vi "FGV Messwerte_PMA.vi"(0 "GasValue":sgl[](array[numeric]), 1 "Messbereich":T2 items=["0-500ppm"=1, "0-2500ppm"=2, "0-10000ppm"=3], 4 "Zielmessbereich":u16, 7 "Prüfgaskonz.":sgl, 8 "Kalibrieren":T4, 9 "Aktion":T5=enum."Messen", 13 "CAL-Daten Tolernaz":T1) -> (14 "Rohwerte LIN":sgl[](array[numeric]), 16 "Rohwerte":sgl[](array[numeric]), 19 "im gültigen Bereich":bool, 20 "GasValue":sgl[](array[numeric]), 21 "CAL-Daten":T3={"O2 Null"=0.0, "O2 Steil"=[1.0, 1.0, 1.0, 1.0]}, 24 "CAL-Daten Tolernaz":T1, 25 "Kalibrieren erfolgreich":bool, 27 "CAL TimeOut":bool)   [LabVIEW 2020, in "ABB-EL3000.lvlib" / "PMA.lvlib" / "Kalibrieren.lvlib"]
uses:
  Kalibrieren.lvlib
  Allgemeine VI/FGV Uras26 Aktion.ctl
  Kalibrierung O2.ctl
  Allgemeine VI/CAL-Daten PMA.ctl
  Allgemeine VI/Messbereich CO lo.ctl
  Allgemeine VI/CAL-Daten Toleranz.ctl
  Auto Kalibrieren/KAL Daten loggen Aktionen.ctl
  Allgemeine VI/Aktionen Cal Daten speichern.ctl
  Allgemein/allgemeine Sub-VIs.lvlib
  Allgemeine VI/Allgemeine VI.lvlib
  Auto Kalibrieren/Auto Kalibrieren.lvlib
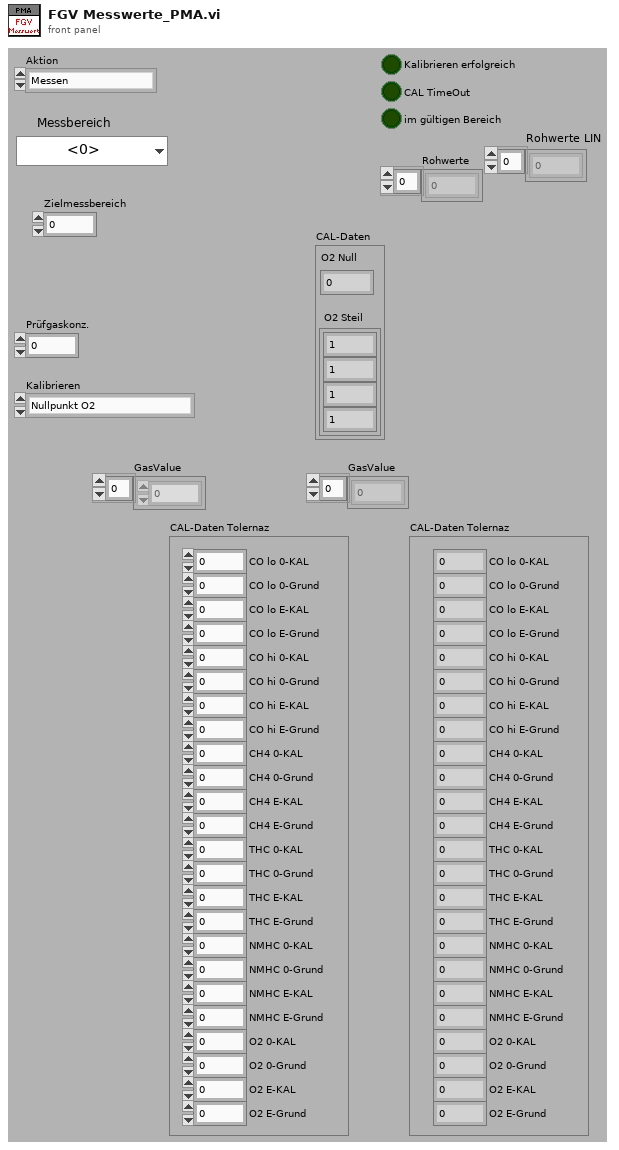
[diagram p1: front panel]
types:
  T1 = typedef "ABB-EL3000.lvlib/Allgemeine VI.lvlib/CAL-Daten Toleranz.ctl" = cluster{"CO lo 0-KAL":sgl, "CO lo 0-Grund":sgl, "CO lo E-KAL":sgl, "CO lo E-Grund":sgl, "CO hi 0-KAL":sgl, "CO hi 0-Grund":sgl, "CO hi E-KAL":sgl, "CO hi E-Grund":sgl, "CH4 0-KAL":sgl, "CH4 0-Grund":sgl, "CH4 E-KAL":sgl, "CH4 E-Grund":sgl, "THC 0-KAL":sgl, "THC 0-Grund":sgl, "THC E-KAL":sgl, "THC E-Grund":sgl, "NMHC 0-KAL":sgl, "NMHC 0-Grund":sgl, "NMHC E-KAL":sgl, "NMHC E-Grund":sgl, "O2 0-KAL":sgl, "O2 0-Grund":sgl, "O2 E-KAL":sgl, "O2 E-Grund":sgl}
  T2 = typedef "ABB-EL3000.lvlib/Allgemeine VI.lvlib/Messbereich CO lo.ctl" = u16
  T3 = typedef "ABB-EL3000.lvlib/Allgemeine VI.lvlib/CAL-Daten PMA.ctl" = cluster{"O2 Null":sgl, "O2 Steil":sgl[]}
  T4 = typedef "ABB-EL3000.lvlib/PMA.lvlib/Kalibrieren.lvlib/Kalibrierung O2.ctl" = enum16{"Nullpunkt O2", "Endpunkt O2"}
  T5 = typedef "ABB-EL3000.lvlib/Allgemeine VI.lvlib/FGV Uras26 Aktion.ctl" = enum16{"lesen", "CAL-Daten laden", "Messen", "Kalibrieren vorbereiten", "Kalibrieren", "CAL-Daten speichern", "Toleranz schreiben", "CAL-Daten kopieren"}
  T6 = typedef "Auto Kalibrieren.lvlib/KAL Daten loggen Aktionen.ctl" = enum16{"lesen", "initialisieren", "loggen"}
  T7 = typedef "ABB-EL3000.lvlib/Allgemeine VI.lvlib/Aktionen Cal Daten speichern.ctl" = enum16{"Cal Daten", "Toleranzen", "PMA", "FID", "Cal Daten PMA", "Cal Daten FID"}
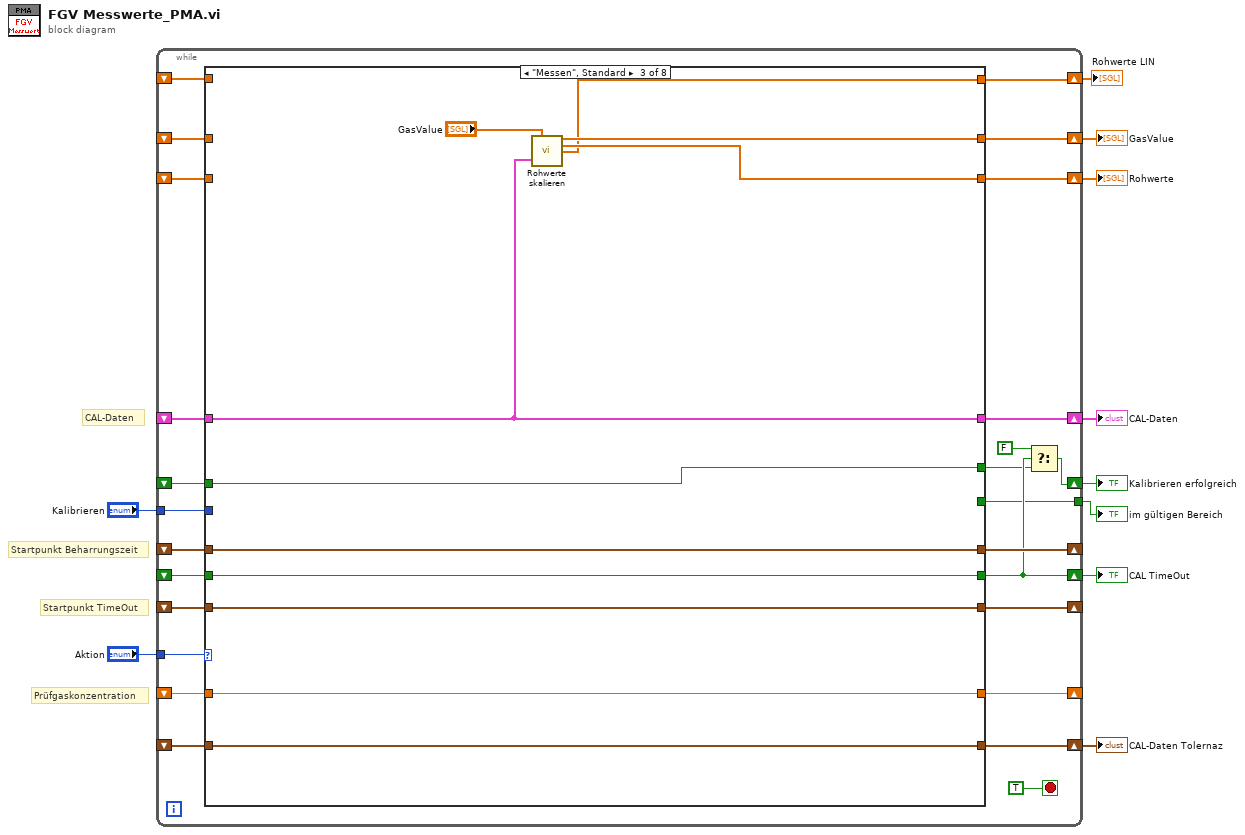
[diagram p0: block diagram]
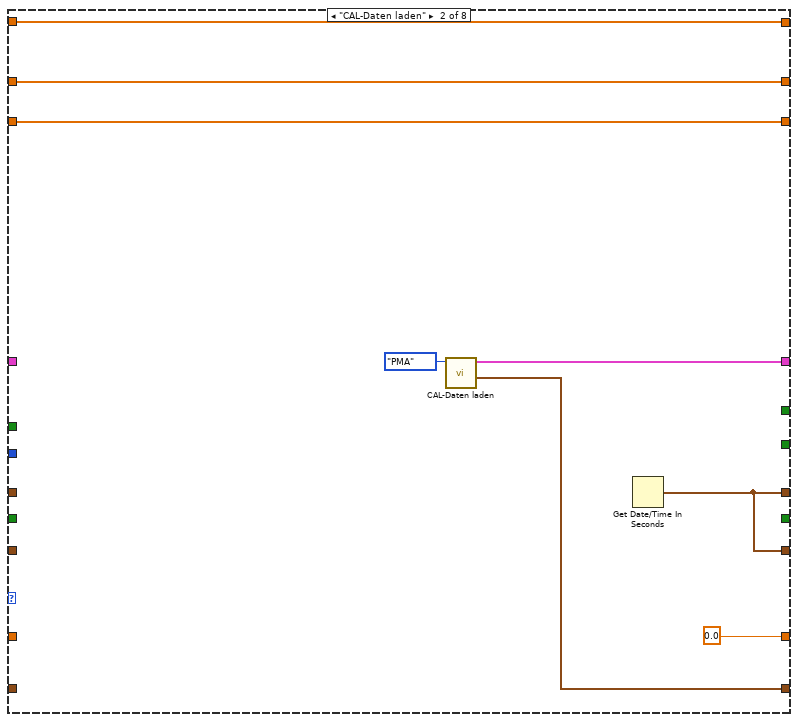
[diagram p3: hidden frame]
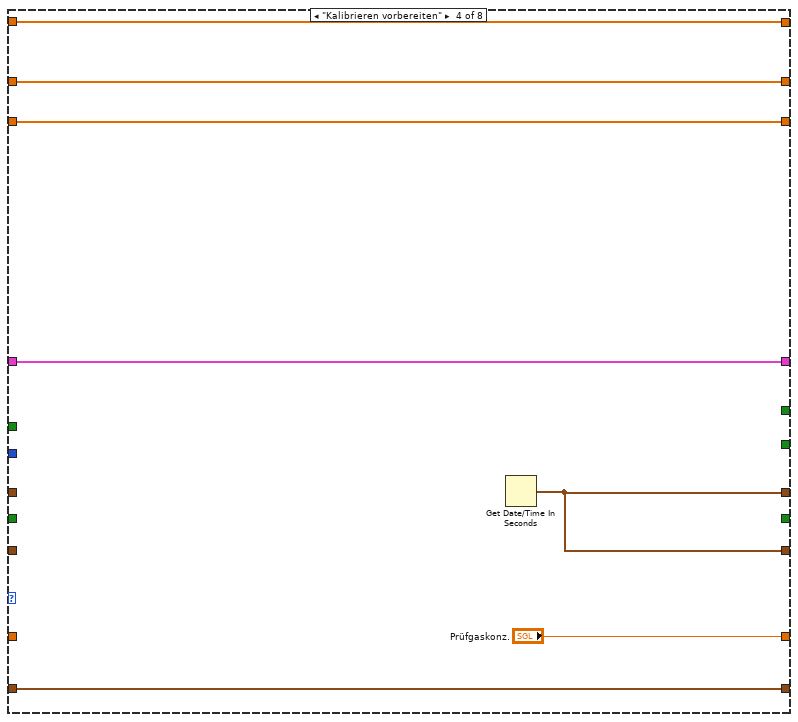
[diagram p4: hidden frame]
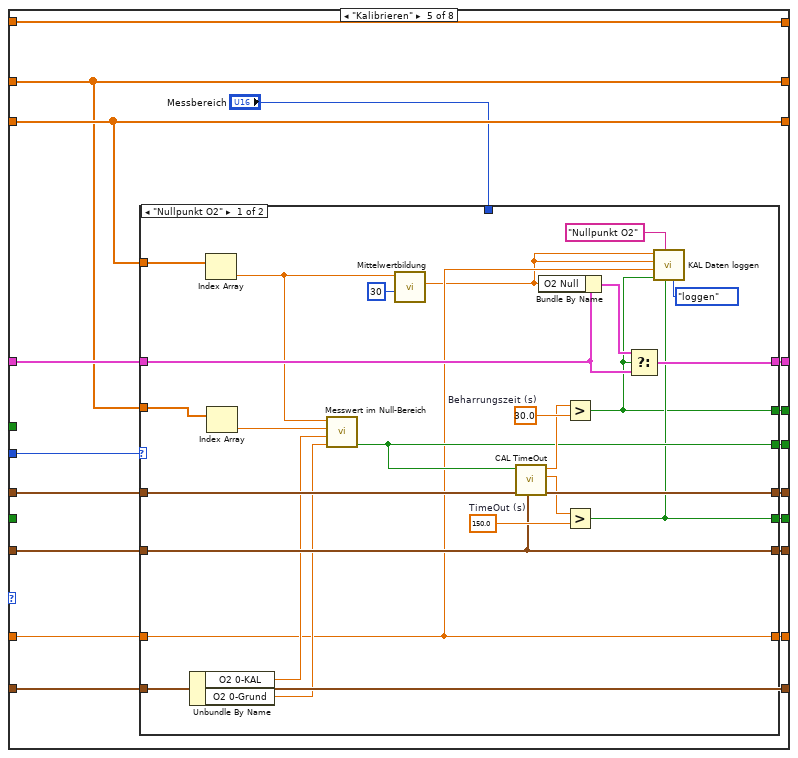
[diagram p5: hidden frame]
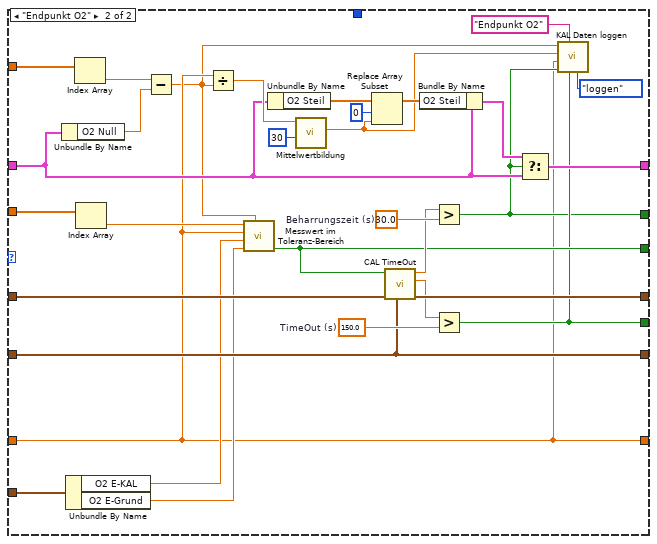
[diagram p6: hidden frame]
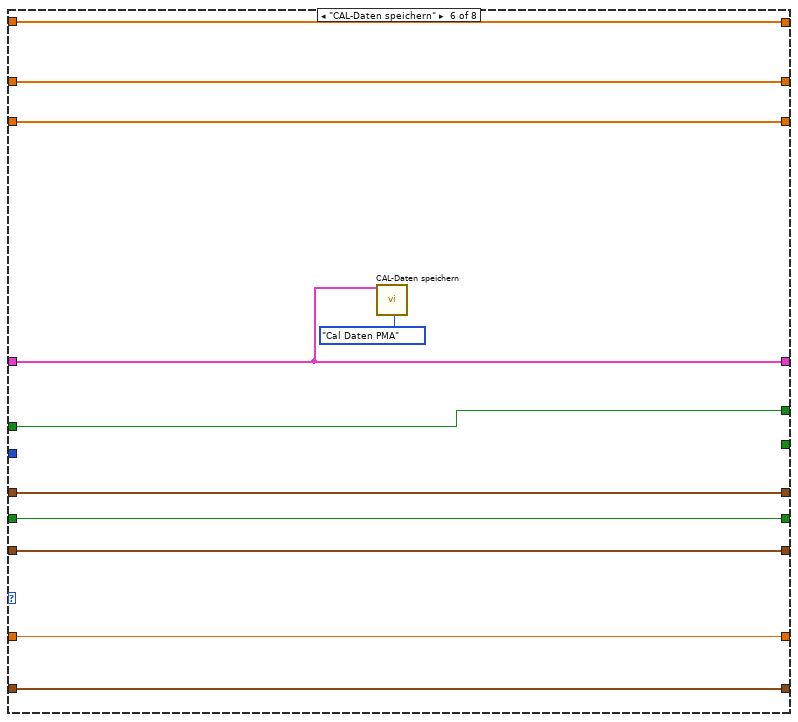
[diagram p7: hidden frame]
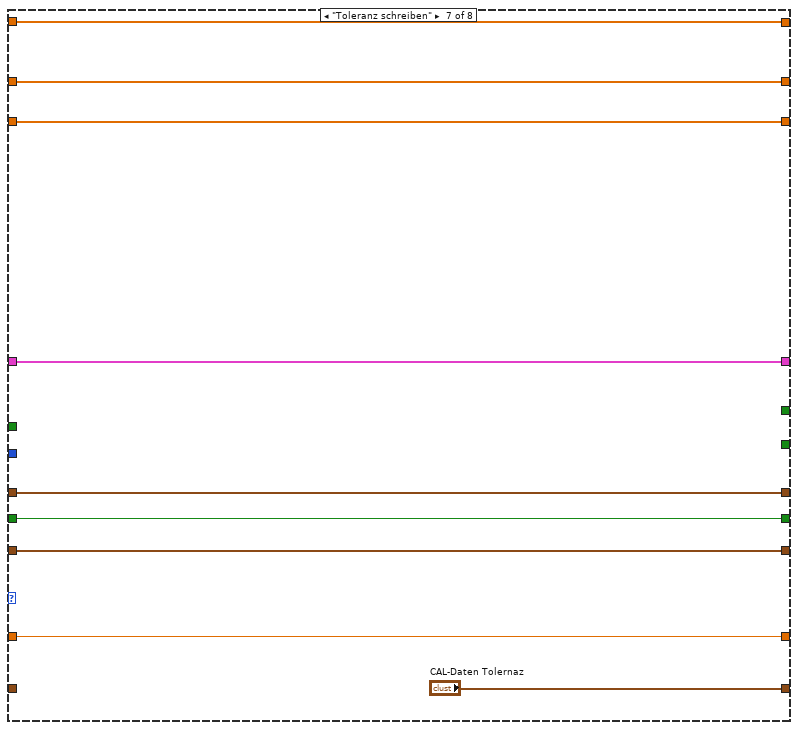
[diagram p8: hidden frame]
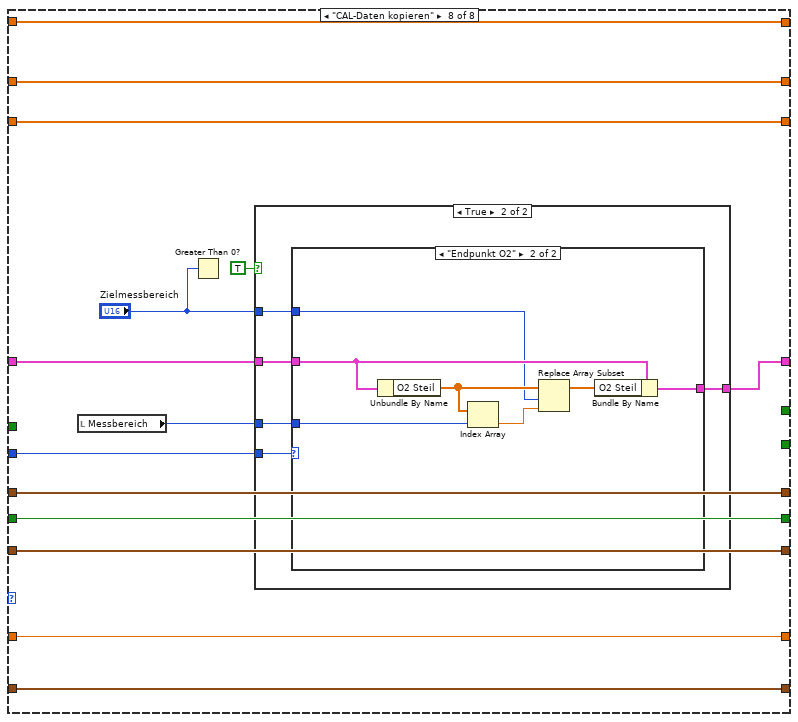
[diagram p9: hidden frame]
diagram:
  # "Prüfgaskonzentration"
  # "Startpunkt TimeOut"
  # "Startpunkt Beharrungszeit"
  # "CAL-Daten"
  n1 = while {
    tunnel: "Aktion" -> [w28]
    shift-right: [w35] -> w6
    shift-left: _ -> [w27]
    tunnel: "Kalibrieren" -> [w34]
    shift-right: [w32] -> _
    shift-left: _ -> [w31]
    shift-right: [w30] -> _
    shift-left: _ -> [w29]
    shift-right: [w22] -> w5
    shift-left: _ -> [w21]
    shift-right: [w24] -> w7
    shift-left: _ -> [w19]
    shift-right: [w26] -> w8
    shift-left: _ -> [w20]
    shift-right: [w18] -> _
    shift-left: _ -> [w33]
    shift-right: [w17] -> w4
    shift-left: _ -> [w16]
    shift-right: [w15] -> w3
    shift-left: _ -> [w14]
    tunnel: [w13] -> w2
    shift-right: [w12] -> w1
    shift-left: _ -> [w11]
    stop <- TRUE stop-if-true
    n2 = case shown="\"Messen\", Standard" w28 {
      tunnel: w27 -> [w44 _ w59 w70 w85 w146 w162 w175]
      tunnel: [w44 w49 w59 w70 w88 w146 w162 w174] -> w35
      tunnel: w34 -> [_ _ _ _ w84 _ _ w176]
      tunnel: w33 -> [w41 _ w60 _ w74 w152 w159 w170]
      tunnel: [w43 w51 w64 w67 w77 w150 w161 w173] -> w32
      tunnel: w31 -> [w43 _ w64 _ w78 w150 w161 w173]
      tunnel: [w42 w51 w63 w67 w75 w149 w160 w171] -> w30
      tunnel: w29 -> [w42 _ w63 _ w76 w149 w160 w171]
      tunnel: [_ _ w61 _ w87 w154 w157 w172] -> w26
      tunnel: [w38 _ w62 _ w86 w153 _ _] -> w25
      tunnel: [w45 w53 w55 w71 w82 w155 w163 w177] -> w22
      tunnel: w21 -> [w45 w53 _ w71 w82 w155 w163 w177]
      tunnel: w20 -> [_ _ w61 _ _ w154 w157 w172]
      tunnel: w19 -> [w38 _ w62 _ _ w153 _ _]
      tunnel: [w41 sgl 0.0 ("Prüfgaskonz.") w60 "Prüfgaskonz." w73 w152 w159 w170] -> w18
      tunnel: [w40 w52 w56 w69 w81 w151 w164 w178] -> w17
      tunnel: w16 -> [w40 w52 _ w69 w81 w151 w164 w178]
      tunnel: [w39 w48 w58 w68 w83 w148 "CAL-Daten Tolernaz" w169] -> w15
      tunnel: w14 -> [w39 _ w58 w68 w83 w148 _ w169]
      tunnel: [_ _ _ _ w79 _ _ _] -> w13
      tunnel: [w37 w46 w54 w65 w72 w145 w156 w165] -> w12
      tunnel: w11 -> [w37 w46 _ w65 w72 w145 w156 w165]
      frame "lesen" {
      }
      frame "CAL-Daten laden" {
        n3 = call "CAL-Daten laden.vi"("Aktion"=enum16{"PMA", "FID"}."PMA") -> ("CAL-Daten Tolernaz"=w48:T1, "CAL-Daten"=w49:T3)  [unwired: 6 in, 3 out]
        n4 = Get Date/Time In Seconds() -> (seconds since 1Jan1904=w51:timestamp)
      }
      frame "Messen", Default {
        n5 = call "Rohwerte skalieren.vi"("GasValue"="GasValue", "CAL-Daten"=w59) -> ("Messwerte"=w56:sgl[], "Rohwerte"=w55:sgl[], "Rohwerte LIN"=w54:sgl[])  [unwired: 11 in]
      }
      frame "Kalibrieren vorbereiten" {
        n6 = Get Date/Time In Seconds() -> (seconds since 1Jan1904=w67:timestamp)
      }
      frame "Kalibrieren" {
        n7 = case shown="\"Nullpunkt O2\"" w84 {
          tunnel: w85 -> [w104 w125]
          tunnel: [w107 w138] -> w88
          tunnel: w74 -> [w90 w116]
          tunnel: w78 -> [w111 w142]
          tunnel: [w109 w140] -> w77
          tunnel: [w110 w141] -> w75
          tunnel: w76 -> [w110 w141]
          tunnel: [w92 w118] -> w87
          tunnel: [w91 w117] -> w86
          tunnel: [w90 w116] -> w73
          tunnel: w83 -> [w102 w132]
          tunnel: w82 -> [w101 w129]
          tunnel: w81 -> [w100 w127]
          tunnel: "Messbereich" -> [_ _]
          tunnel: [w96 w126] -> w79
          frame "Nullpunkt O2" {
            w112 = sgl 150.0  # TimeOut (s)
            w113 = sgl 30.0  # Beharrungszeit (s)
            n8 = Unbundle By Name(w102) -> ("O2 0-KAL"=w98:sgl, "O2 0-Grund"=w97:sgl)
            n9 = Index Array(array=w101) -> (element=w95:sgl)  [unwired: 1 in]
            n10 = Index Array(array=w100) -> (element=w99:sgl)  [unwired: 1 in]
            n11 = call "Messwert im Null-Bereich.vi"("Toleranz Grundkalibrierung"=w97, "Toleranz letzte KAL"=w98, "Messwert"=w99, "Rohwert"=w95) -> ("im Bereich"=w96:bool)  [unwired: 7 in]
            n12 = call "Mittelwertbildung.vi"("Anzahl Werte"=u8 30, "Neuer Wert"=w95) -> ("gemittelter Wert"=w89:sgl)  [unwired: 7 in, 2 out]
            n13 = call "CAL TimeOut.vi"("CAL-Start"=w110, "im Bereich seit"=w111, "im Bereich"=w96) -> ("im Bereich seit (Ausgang)"=w109:timestamp, "Sekunden seit CAL-Start"=w108:sgl, "Sekunden im Bereich"=w106:sgl)  [unwired: 5 in]
            n14 = Bundle By Name(cluster=w104, "O2 Null"=w89) -> (w105:T3)
            n15 = Greater?(x=w106, y=w113) -> (0:w91:bool)
            n16 = Greater?(x=w108, y=w112) -> (0:w92:bool)
            n17 = Select(t=w105, s=w91, f=w104) -> (s? t:f=w107:T3)
            n18 = call "KAL Daten loggen.vi"("Aktionen MFC loggen"=KAL_Daten_loggen_Aktionen."loggen", "TimeOUT"=w92, "Komponente"="Nullpunkt O2", "Kalibrieren Erfolgreich"=w91, "Prüfgaskonzentration"=w90, "Kalibrierwert"=w89, "Rohwert"=w89) -> ()  [unwired: 4 in, 1 out]
          }
          frame "Endpunkt O2" {
            w143 = sgl 150.0  # TimeOut (s)
            w144 = sgl 30.0  # Beharrungszeit (s)
            n19 = Unbundle By Name(w125) -> ("O2 Null"=w123:sgl)
            n20 = Unbundle By Name(w132) -> ("O2 E-KAL"=w131:sgl, "O2 E-Grund"=w130:sgl)
            n21 = Index Array(array=w129) -> (element=w124:sgl)  [unwired: 1 in]
            n22 = Index Array(array=w127) -> (element=w128:sgl)  [unwired: 1 in]
            n23 = Subtract(x=w124, y=w123) -> (x-y=w114:sgl)
            n24 = Divide(x=w116, y=w114) -> (x/y=w133:sgl)
            n25 = call "Messwert im Toleranz-Bereich.vi"("Rohwert"=w114, "Toleranz Grundkalibrierung"=w130, "Toleranz in % letzte KAL"=w131, "Prüfgas-Konzentration"=w116, "Messwert"=w128) -> ("im Bereich"=w126:bool)  [unwired: 6 in]
            n26 = Unbundle By Name(w125) -> ("O2 Steil"=w136:sgl[])
            n27 = call "Mittelwertbildung.vi"("Anzahl Werte"=u8 30, "Neuer Wert"=w133) -> ("gemittelter Wert"=w115:sgl)  [unwired: 7 in, 2 out]
            n28 = Replace Array Subset(array=w136, new element=w115, index=0 ("Index")) -> (w135:sgl[])
            n29 = call "CAL TimeOut.vi"("CAL-Start"=w141, "im Bereich seit"=w142, "im Bereich"=w126) -> ("im Bereich seit (Ausgang)"=w140:timestamp, "Sekunden seit CAL-Start"=w139:sgl, "Sekunden im Bereich"=w137:sgl)  [unwired: 5 in]
            n30 = Bundle By Name(cluster=w125, "O2 Steil"=w135) -> (w122:T3)
            n31 = Greater?(x=w137, y=w144) -> (0:w117:bool)
            n32 = Greater?(x=w139, y=w143) -> (0:w118:bool)
            n33 = Select(t=w122, s=w117, f=w125) -> (s? t:f=w138:T3)
            n34 = call "KAL Daten loggen.vi"("Aktionen MFC loggen"=KAL_Daten_loggen_Aktionen."loggen", "TimeOUT"=w118, "Komponente"="Endpunkt O2", "Kalibrieren Erfolgreich"=w117, "Prüfgaskonzentration"=w116, "Kalibrierwert"=w115, "Rohwert"=w114) -> ()  [unwired: 4 in, 1 out]
          }
        }
      }
      frame "CAL-Daten speichern" {
        n35 = call "CAL-Daten speichern.vi"("CAL-Daten PMA"=w146, "Aktionen Kal Daten speichern"=Aktionen_Cal_Daten_speichern."Cal Daten PMA") -> ()  [unwired: 18 in]
      }
      frame "Toleranz schreiben" {
      }
      frame "CAL-Daten kopieren" {
        n36 = local read "Messbereich"() -> (w167:T2)
        n37 = Greater Than 0?(x="Zielmessbereich") -> ()  [unwired: 1 out]
        n38 = case shown="True" TRUE {
          tunnel: w176 -> [_ w184]
          tunnel: w175 -> [w179 w183]
          tunnel: w167 -> [_ w182]
          tunnel: [w179 w181] -> w174
          tunnel: "Zielmessbereich" -> [_ w180]
          frame False {
          }
          frame True {
            n39 = case shown="\"Endpunkt O2\"" w184 {
              tunnel: w183 -> [w185 w191]
              tunnel: w182 -> [_ w189]
              tunnel: w180 -> [_ w187]
              tunnel: [w185 w186] -> w181
              frame "Nullpunkt O2", Default {
              }
              frame "Endpunkt O2" {
                n40 = Unbundle By Name(w191) -> ("O2 Steil"=w190:sgl[])
                n41 = Index Array(array=w190, index=w189) -> (element=w188:sgl)
                n42 = Replace Array Subset(array=w190, new element=w188, index=w187) -> (w192:sgl[])
                n43 = Bundle By Name(cluster=w191, "O2 Steil"=w192) -> (w186:T3)
              }
            }
          }
        }
      }
    }
    n44 = Select(t=FALSE, s=w26, f=w25) -> (s? t:f=w24:bool)
  }
  "Kalibrieren erfolgreich" <- w7
  "CAL TimeOut" <- w8
  "CAL-Daten" <- w6
  "Rohwerte" <- w5
  "GasValue" <- w4
  "CAL-Daten Tolernaz" <- w3
  "im gültigen Bereich" <- w2
  "Rohwerte LIN" <- w1
